vi "02.4 Acquire Data (subVI).vi"(8 "Error In":errorcluster, 11 "physical channels":tag) -> (0 "error out":errorcluster, 3 "2D DBL":dbl[][](array[numeric]))   [LabVIEW 2019]
uses:
  02.4 DAQmx Configuration Cluster.ctl
  <vilib>/DAQmx/read.llb/DAQmx Read (Analog 2D DBL NChan NSamp).vi
  <vilib>/DAQmx/create/channels.llb/DAQmx Create Channel (AI-Voltage-Basic).vi
  <vilib>/DAQmx/configure/timing.llb/DAQmx Timing (Sample Clock).vi
  <vilib>/DAQmx/miscellaneous.llb/DAQmx Fill In Error Info.vi
panel:
  in  "DAQmx Configuration Cluster":T1={"Desired Sample Rate (Hz)"=-1.0, "sample mode"=10178, "Minimum value"=-1.0, "Maximum value"=-1.0, "Physical Channel"="", "units"=10143, "thermocouple type"=10072, "Samples per Channel"=0} {"thermocouple type" items=["J"=10072, "K"=10073, "N"=10077, "R"=10082, "S"=10085, "T"=10086, "B"=10047, "E"=10055]; "units" items=["Deg C"=10143, "Deg F"=10144, "Kelvins"=10325, "Deg R"=10145, "From Custom Scale"=10065]; "sample mode" items=["Finite Samples"=10178, "Continuous Samples"=10123, "Hardware Timed Single Point"=12522]}
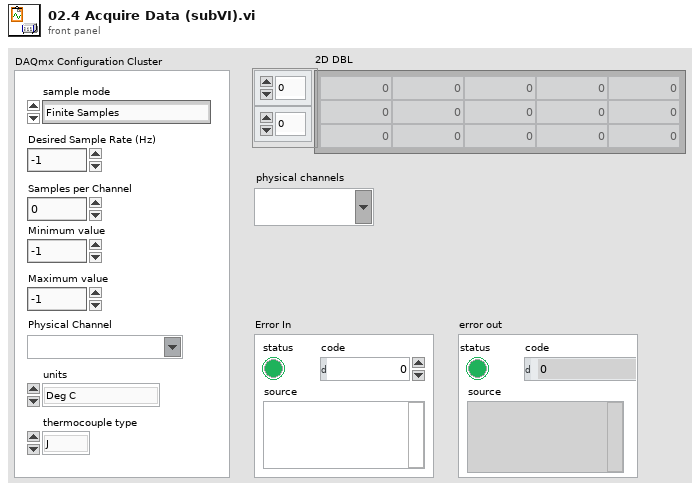
[diagram p1: front panel]
types:
  T1 = typedef "02.4 DAQmx Configuration Cluster.ctl" = cluster{"Desired Sample Rate (Hz)":dbl, "sample mode":i32, "Minimum value":dbl, "Maximum value":dbl, "Physical Channel":tag, "units":i32, "thermocouple type":i32, "Samples per Channel":i32}
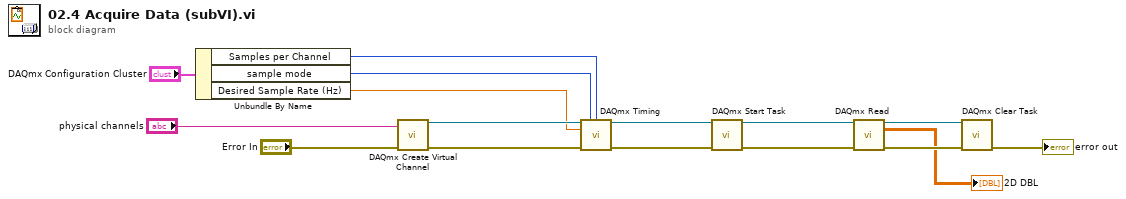
[diagram p0: block diagram]
diagram:
  n1 = Unbundle By Name("DAQmx Configuration Cluster") -> ("Samples per Channel"=w2:i32, "sample mode"=w3:i32, "Desired Sample Rate (Hz)"=w4:dbl)
  n2 = call-poly <vilib>:"DAQmx Create Virtual Channel.vi"("physical channels"="physical channels", "error in"="Error In") -> ("task out"=w15:refnum<k21>, "error out"=w16:errorcluster)  [unwired: 12 in]
  n3 = call-poly <vilib>:"DAQmx Timing.vi"("task/channels in"=w15, "sample mode"=w3, "samples per channel"=w2, "rate"=w4, "error in"=w16) -> ("task out"=w9:refnum<k21>, "error out"=w10:errorcluster)  [unwired: 9 in]
  n4 = call <vilib>:"DAQmx Start Task.vi"("task/channels in"=w9, "error in"=w10) -> ("task out"=w11:refnum<k21>, "error out"=w12:errorcluster)  [unwired: 12 in]
  n5 = call-poly <vilib>:"DAQmx Read.vi"("task/channels in"=w11, "error in"=w12) -> ("task out"=w14:refnum<k21>, "data"=→"2D DBL":dbl[][], "error out"=w13:errorcluster)  [unwired: 11 in]
  n6 = call <vilib>:"DAQmx Clear Task.vi"("task in"=w14, "error in"=w13) -> ("error out"=→"error out":errorcluster)  [unwired: 13 in]
